vi "Find Object.vi"(8 "error in (no error)":errorcluster, 10 "Object Name":string, 11 "Scene Refnum":refnum<vi>) -> (0 "error out":errorcluster, 3 "Object Refnum":refnum<vi>)   [LabVIEW 2020, in "NI_3D Picture Control.lvlib"]
doc: "Takes a 3D scene reference and an object name and returns the first object in the scene with a matching name."
uses:
  <vilib>/picture/3D Picture Control/NI_3D Picture Control.lvlib
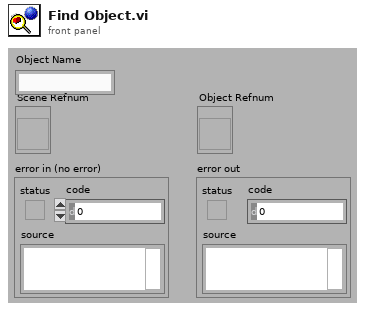
[diagram p1: front panel]
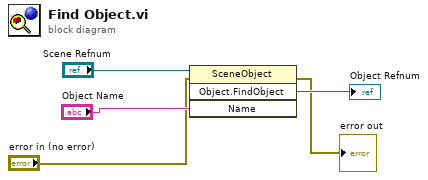
[diagram p0: block diagram]
diagram:
  n1 = invoke class="SceneObject" method="Object.FindObject"(reference="Scene Refnum", error in="error in (no error)", "Name"="Object Name") -> (error out=→"error out":errorcluster, "FindObject"=→"Object Refnum":refnum<vi>)  [unwired: 1 in, 2 out]
